vi "Item_OnCommand.vi"(10 "Command ID":string, 11 "Object":T1) -> ()   [LabVIEW 2020, in "Triarc Project Provider.lvlib"]
uses:
  Triarc Project Provider.lvlib
  <resource>/Framework/Providers/API/ItemRef.ctl
panel:
  out "error out":errorcluster
  in  "error in":errorcluster
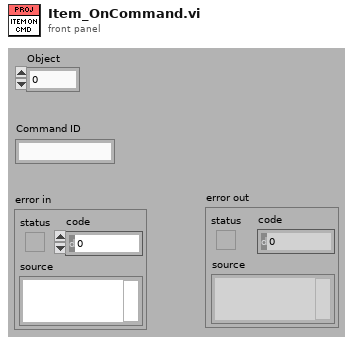
[diagram p1: front panel]
types:
  T1 = typedef "ItemRef.ctl" = u64
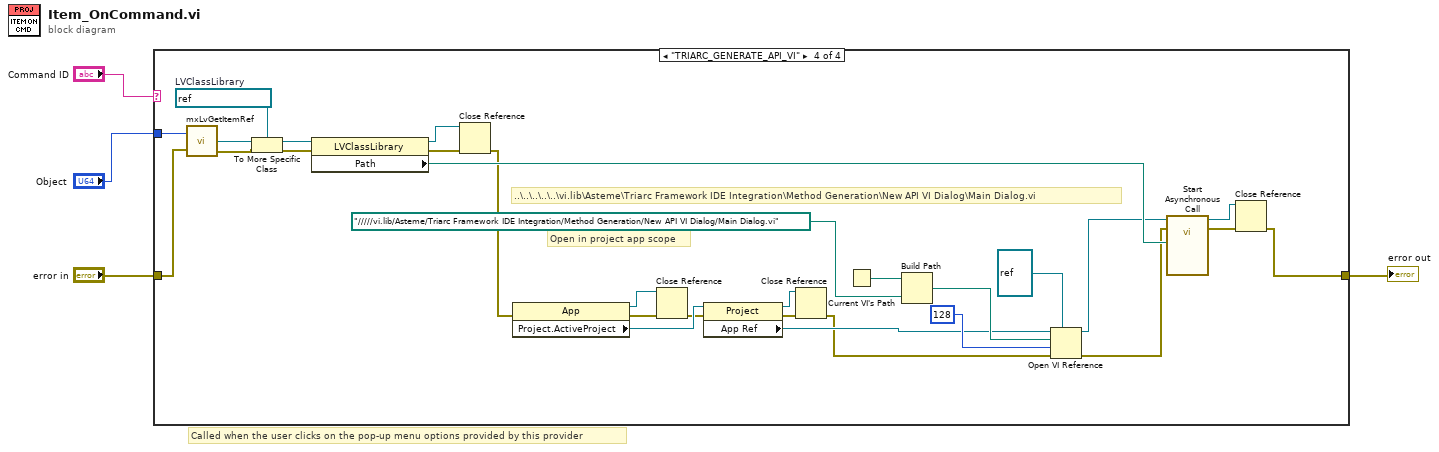
[diagram p0: block diagram]
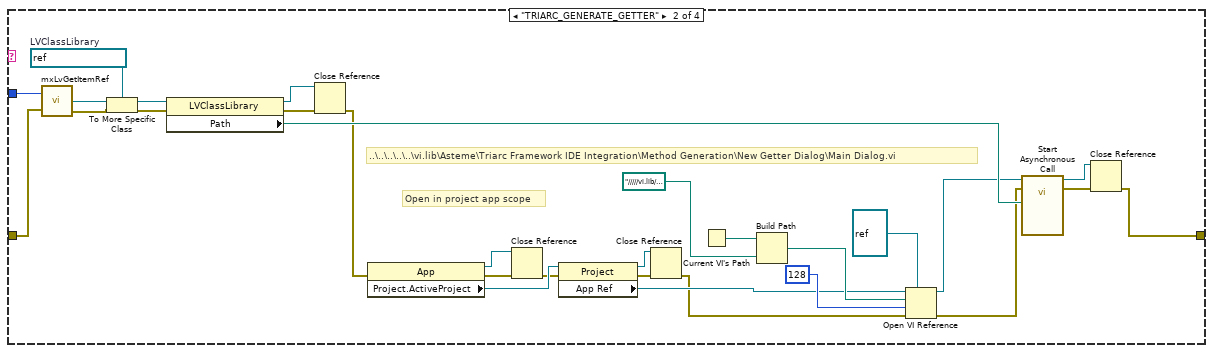
[diagram p3: hidden frame]
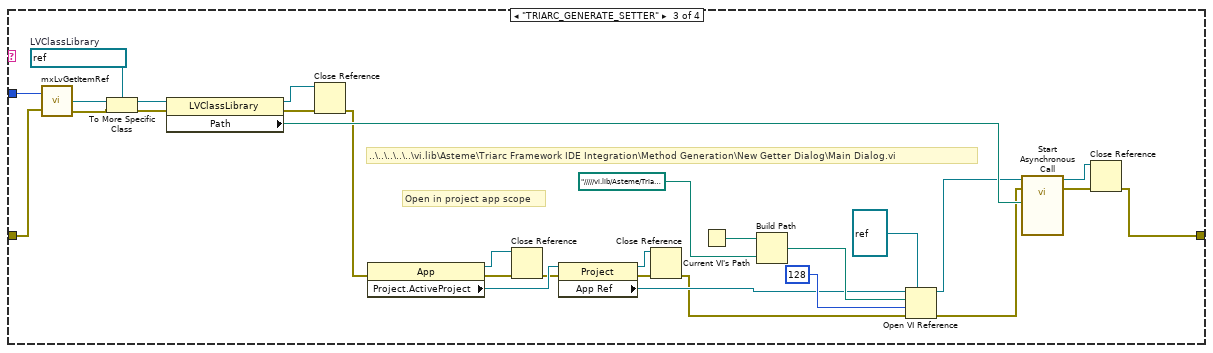
[diagram p4: hidden frame]
diagram:
  # "Called when the user clicks on the pop-up menu options provided by this provider"
  n1 = case shown="\"TRIARC_GENERATE_API_VI\"" "Command ID" {
    tunnel: "error in" -> [w5 w33 w62 w91]
    tunnel: [w5 w7 w36 w65] -> w2
    tunnel: "Object" -> [_ w34 w63 w92]
    frame Default {
    }
    frame "TRIARC_GENERATE_GETTER" {
      w30 = refnum<vi> refnum  # LVClassLibrary
      # "..\\..\\..\\..\\..\\vi.lib\\Asteme\\Triarc Framework IDE Integration\\Method Generation\\New Getter Dialog\\Main Dialog.vi"
      # "Open in project app scope"
      n2 = call <resource>:"mxLvGetItemRef.vi"("Item"=w34, "error in"=w33) -> ("Item Refnum"=w32:refnum<vi>, "error out"=w23:errorcluster)  [unwired: 1 out]
      n3 = To More Specific Class(target class=w30, reference=w32, error in=w23) -> (specific class reference=w31:refnum<vi>, error out=w29:errorcluster)
      n4 = property class="LVClassLibrary"(reference=w31, error in=w29) -> (reference out=w27:refnum<vi>, error out=w28:errorcluster, "Path"=w25:path)
      n5 = Close Reference(reference=w27, error in (no error)=w28) -> (error out=w19:errorcluster)
      n6 = property class="App"(error in=w19) -> (reference out=w9:refnum<vi>, error out=w11:errorcluster, "Project.ActiveProject"=w16:refnum<vi>)  [unwired: 1 in]
      n7 = Close Reference(reference=w9, error in (no error)=w11) -> (error out=w10:errorcluster)
      n8 = property class="Project"(reference=w16, error in=w10) -> (reference out=w15:refnum<vi>, error out=w13:errorcluster, "App Ref"=w14:refnum<vi>)
      n9 = Close Reference(reference=w15, error in (no error)=w13) -> (error out=w12:errorcluster)
      n10 = Current VI's Path() -> (path=w17:path)
      n11 = Build Path(base path=w17, name or relative path=path "../../../../../vi.lib/Asteme/Triarc Framework IDE Integration/Method Generation/New Getter Dialog/Main Dialog.vi" ("Relative Path from 1 to 2")) -> (appended path=w22:path)
      n12 = Open VI Reference(type specifier VI Refnum (for type only)=refnum<vi> refnum, application reference (local)=w14, vi path=w22, options=128, error in (no error)=w12) -> (vi reference=w21:refnum<vi>, error out=w8:errorcluster)  [unwired: 1 in]
      n13 = call-by-ref "Start Asynchronous Call"(reference=w21, error in=w8, "Process Path"=w25) -> (reference out=w24:refnum<vi>, error out=w26:errorcluster)  [unwired: 11 in]
      n14 = Close Reference(reference=w24, error in (no error)=w26) -> (error out=w7:errorcluster)
    }
    frame "TRIARC_GENERATE_SETTER" {
      w59 = refnum<vi> refnum  # LVClassLibrary
      # "..\\..\\..\\..\\..\\vi.lib\\Asteme\\Triarc Framework IDE Integration\\Method Generation\\New Getter Dialog\\Main Dialog.vi"
      # "Open in project app scope"
      n15 = call <resource>:"mxLvGetItemRef.vi"("Item"=w63, "error in"=w62) -> ("Item Refnum"=w61:refnum<vi>, "error out"=w52:errorcluster)  [unwired: 1 out]
      n16 = To More Specific Class(target class=w59, reference=w61, error in=w52) -> (specific class reference=w60:refnum<vi>, error out=w58:errorcluster)
      n17 = property class="LVClassLibrary"(reference=w60, error in=w58) -> (reference out=w56:refnum<vi>, error out=w57:errorcluster, "Path"=w54:path)
      n18 = Close Reference(reference=w56, error in (no error)=w57) -> (error out=w48:errorcluster)
      n19 = property class="App"(error in=w48) -> (reference out=w38:refnum<vi>, error out=w40:errorcluster, "Project.ActiveProject"=w45:refnum<vi>)  [unwired: 1 in]
      n20 = Close Reference(reference=w38, error in (no error)=w40) -> (error out=w39:errorcluster)
      n21 = property class="Project"(reference=w45, error in=w39) -> (reference out=w44:refnum<vi>, error out=w42:errorcluster, "App Ref"=w43:refnum<vi>)
      n22 = Close Reference(reference=w44, error in (no error)=w42) -> (error out=w41:errorcluster)
      n23 = Current VI's Path() -> (path=w46:path)
      n24 = Build Path(base path=w46, name or relative path=path "../../../../../vi.lib/Asteme/Triarc Framework IDE Integration/Method Generation/New Setter Dialog/Main Dialog.vi" ("Relative Path from 1 to 2")) -> (appended path=w51:path)
      n25 = Open VI Reference(type specifier VI Refnum (for type only)=refnum<vi> refnum, application reference (local)=w43, vi path=w51, options=128, error in (no error)=w41) -> (vi reference=w50:refnum<vi>, error out=w37:errorcluster)  [unwired: 1 in]
      n26 = call-by-ref "Start Asynchronous Call"(reference=w50, error in=w37, "Process Path"=w54) -> (reference out=w53:refnum<vi>, error out=w55:errorcluster)  [unwired: 11 in]
      n27 = Close Reference(reference=w53, error in (no error)=w55) -> (error out=w36:errorcluster)
    }
    frame "TRIARC_GENERATE_API_VI" {
      w88 = refnum<vi> refnum  # LVClassLibrary
      # "..\\..\\..\\..\\..\\vi.lib\\Asteme\\Triarc Framework IDE Integration\\Method Generation\\New API VI Dialog\\Main Dialog.vi"
      # "Open in project app scope"
      n28 = call <resource>:"mxLvGetItemRef.vi"("Item"=w92, "error in"=w91) -> ("Item Refnum"=w90:refnum<vi>, "error out"=w81:errorcluster)  [unwired: 1 out]
      n29 = To More Specific Class(target class=w88, reference=w90, error in=w81) -> (specific class reference=w89:refnum<vi>, error out=w87:errorcluster)
      n30 = property class="LVClassLibrary"(reference=w89, error in=w87) -> (reference out=w85:refnum<vi>, error out=w86:errorcluster, "Path"=w83:path)
      n31 = Close Reference(reference=w85, error in (no error)=w86) -> (error out=w77:errorcluster)
      n32 = property class="App"(error in=w77) -> (reference out=w67:refnum<vi>, error out=w69:errorcluster, "Project.ActiveProject"=w74:refnum<vi>)  [unwired: 1 in]
      n33 = Close Reference(reference=w67, error in (no error)=w69) -> (error out=w68:errorcluster)
      n34 = property class="Project"(reference=w74, error in=w68) -> (reference out=w73:refnum<vi>, error out=w71:errorcluster, "App Ref"=w72:refnum<vi>)
      n35 = Close Reference(reference=w73, error in (no error)=w71) -> (error out=w70:errorcluster)
      n36 = Current VI's Path() -> (path=w75:path)
      n37 = Build Path(base path=w75, name or relative path=path "../../../../../vi.lib/Asteme/Triarc Framework IDE Integration/Method Generation/New API VI Dialog/Main Dialog.vi" ("Relative Path from 1 to 2")) -> (appended path=w80:path)
      n38 = Open VI Reference(type specifier VI Refnum (for type only)=refnum<vi> refnum, application reference (local)=w72, vi path=w80, options=128, error in (no error)=w70) -> (vi reference=w79:refnum<vi>, error out=w66:errorcluster)  [unwired: 1 in]
      n39 = call-by-ref "Start Asynchronous Call"(reference=w79, error in=w66, "Process Path"=w83) -> (reference out=w82:refnum<vi>, error out=w84:errorcluster)  [unwired: 11 in]
      n40 = Close Reference(reference=w82, error in (no error)=w84) -> (error out=w65:errorcluster)
    }
  }
  "error out" <- w2
